vi "DeferPanelUpdates.vi"(8 "error in":errorcluster, 10 "deferPanelUpdates in":bool, 11 "VI in":refnum<vi>) -> (0 "error out":errorcluster, 3 "VI out":refnum<vi>)   [LabVIEW 2010, in "StyledText.lvlib"]
doc: "Wraps the property setting 'DeferPanelUpdates' of the frontpanel belonging to <b>VI</b>.\n\nCopyright (c) 2018, Martin Weiss\nAll rights reserved.\n\nRedistribution and use in source and binary forms, with or without modification, are permitted provided that the following conditions are met:\n\n1. Redistributions of source code must retain the above copyright notice, this list of conditions and the following disclaimer.\n\n2. Redistributions in binary form must reproduce the above copyright notice, this list of conditions and the following disclaimer in the documentation and/or other materials provided with the distribution.\n\nTHIS SOFTWARE IS PROVIDED BY THE COPYRIGHT HOLDERS AND CONTRIBUTORS \"AS IS\" AND ANY EXPRESS OR IMPLIED WARRANTIES, INCLUDING, BUT NOT LIMITED TO, THE IMPLIED WARRANTIES OF MERCHANTABILITY AND FITNESS FOR A PARTICULAR PURPOSE ARE DISCLAIMED. IN NO EVENT SHALL THE COPYRIGHT HOLDER OR CONTRIBUTORS BE LIABLE FOR ANY DIRECT, INDIRECT, INCIDENTAL, SPECIAL, EXEMPLARY, OR CONSEQUENTIAL DAMAGES (INCLUDING, BUT NOT LIMITED TO, PROCUREMENT OF SUBSTITUTE GOODS OR SERVICES; LOSS OF USE, DATA, OR PROFITS; OR BUSINESS INTERRUPTION) HOWEVER CAUSED AND ON ANY THEORY OF LIABILITY, WHETHER IN CONTRACT, STRICT LIABILITY, OR TORT (INCLUDING NEGLIGENCE OR OTHERWISE) ARISING IN ANY WAY OUT OF THE USE OF THIS SOFTWARE, EVEN IF ADVISED OF THE POSSIBILITY OF SUCH DAMAGE."
uses:
  StyledText.lvlib
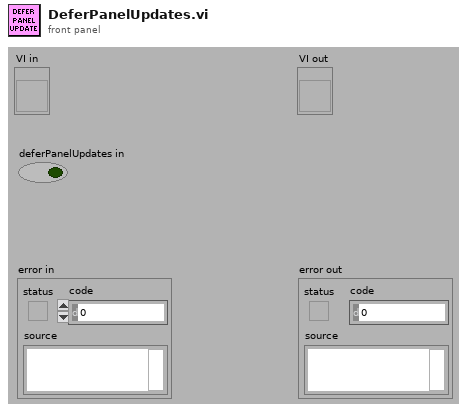
[diagram p1: front panel]
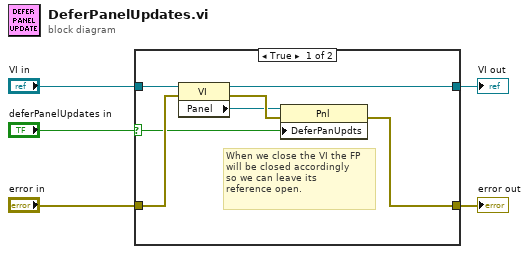
[diagram p0: block diagram]
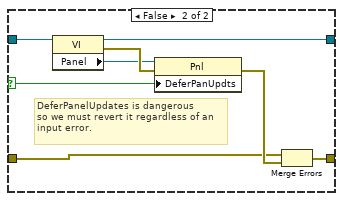
[diagram p2: hidden frame]
diagram:
  n1 = case shown="True" "deferPanelUpdates in" {
    selector: "deferPanelUpdates in" -> [w6 w15]
    tunnel: [w12 w14] -> w5
    tunnel: "error in" -> [w10 w13]
    tunnel: [w8 w17] -> w3
    tunnel: "VI in" -> [w7 w16]
    frame True {
      # "When we close the VI the FP\nwill be closed accordingly\nso we can leave its\nreference open."
      n2 = property class="VI"(reference=w7, error in=w10) -> (reference out=w8:refnum<vi>, error out=w11:errorcluster, "Panel"=w9:refnum<vi>)
      n3 = property class="Pnl"(reference=w9, error in=w11, "DeferPanUpdts"=w6) -> (error out=w12:errorcluster)  [unwired: 1 out]
    }
    frame False {
      # "DeferPanelUpdates is dangerous\nso we must revert it regardless of an\ninput error."
      n4 = property class="VI"(reference=w16) -> (reference out=w17:refnum<vi>, error out=w19:errorcluster, "Panel"=w18:refnum<vi>)  [unwired: 1 in]
      n5 = property class="Pnl"(reference=w18, error in=w19, "DeferPanUpdts"=w15) -> (error out=w20:errorcluster)  [unwired: 1 out]
      n6 = Merge Errors(w13, w20) -> (w14:errorcluster)
    }
  }
  "error out" <- w5
  "VI out" <- w3
